vi "Pendulum7_0.vi"() -> ()   [LabVIEW 2021]
uses:
  <vilib>/Utility/miscctls.llb/LVBoundsTypeDef.ctl
  <vilib>/Platform/TimedLoop/XDataNode/timing_clust.ctl
  <vilib>/Platform/TimedLoop/XDataNode/nitl_modes.ctl
  <vilib>/Platform/TimedLoop/XDataNode/wakeup.ctl
  <vilib>/platform/TimedLoop/XDataNode/XDataNode.xnode
  <vilib>/Platform/TimedLoop/XDataNode/XDNodeRunTimeDep.lvlib
panel:
  out "error out":errorcluster
  in  "Enum 2":enum16{"stop", "start"}(ring)
  out "L":dbl
  out "Waveform Graph 2":waveform(dbl)(graph)
  in  "Остановить симуляцию":bool
  in  "Начать симуляцию":bool
  out "Object":bool
  in  "Cieling":bool
  in  "Начальная амплитуда":dbl
  in  "Амплитуда":dbl
  in  "Угловая частота внешней силы":dbl min=0.0
  in  "Вязкость среды":dbl min=0.0
  in  "Масса":dbl min=0.0 max=3000.0
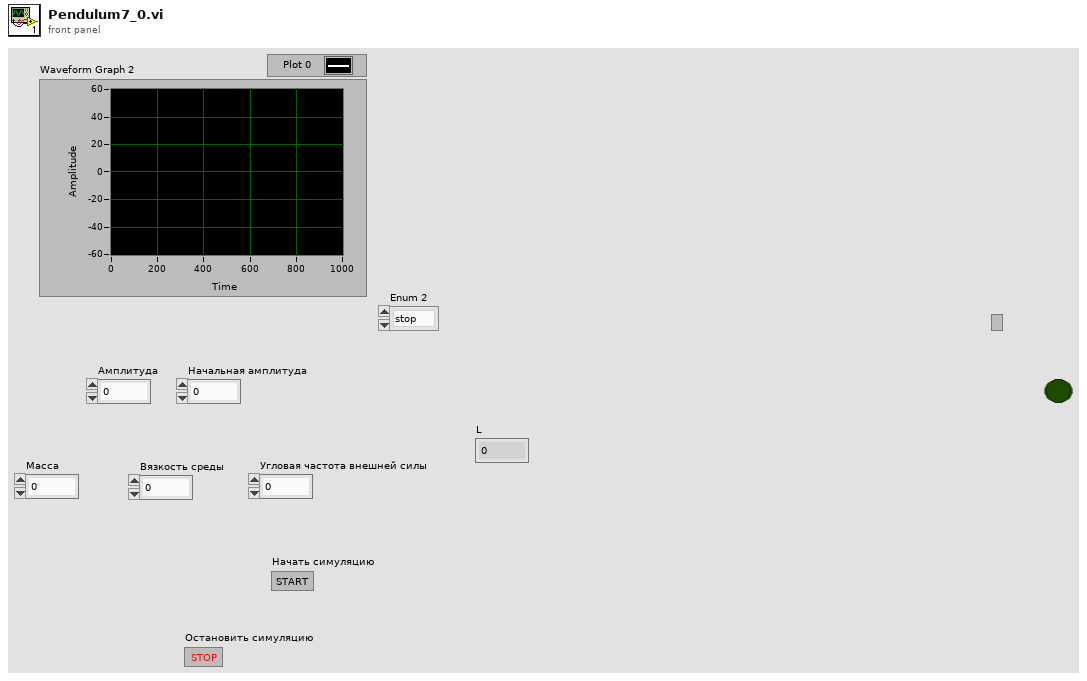
[diagram p1: front panel]
types:
  T1 = typedef "XDNodeRunTimeDep.lvlib/timing_clust.ctl" = cluster{"Expected End [f-1]":u64, "Actual End [f-1]":u64, "Finished Late? [f-1]":bool, "Expected End [i-1]":u64, "Actual End [i-1]":u64, "Finished Late? [i-1]":bool, "Expected Start [i]":u64, "Actual Start [i]":u64, "Expected Start [f]":u64, "Actual Start [f]":u64, "Source Name":string, "Structure Name":string, "Period":i64, "Deadline":i64, "Offset":i64, "Start":i64, "Priority":i32, "Timeout":i32, "Mode":T2, "Wakeup Reason":T3, "Error":errorcluster, "Source Type":string, "Secondary Source Type":string, "Global End Time":u64, "Global Start Time":u64, "Frame Duration":u64, "Iteration Duration":u64, "Assigned CPU":i32, "I/O Scan Engine Mode":u32}
  T2 = typedef "XDNodeRunTimeDep.lvlib/nitl_modes.ctl" = enum32{"No Change", "Process missed periods, maintain original phase", "Discard missed periods, maintain original phase", "Process missed periods, ignore original phase", "Discard missed periods, ignore original phase"}
  T3 = typedef "XDNodeRunTimeDep.lvlib/wakeup.ctl" = enum32{"Normal", "Aborted", "Asynchronous wakeup", "Timing source error", "Timed loop error", "Timeout"}
  T4 = typedef "LVBoundsTypeDef.ctl" = cluster{"Width":u32, "Height":u32}
  T5 = typedef "LVPoint32TypeDef.ctl" = cluster{"Horizontal":i32, "Vertical":i32}
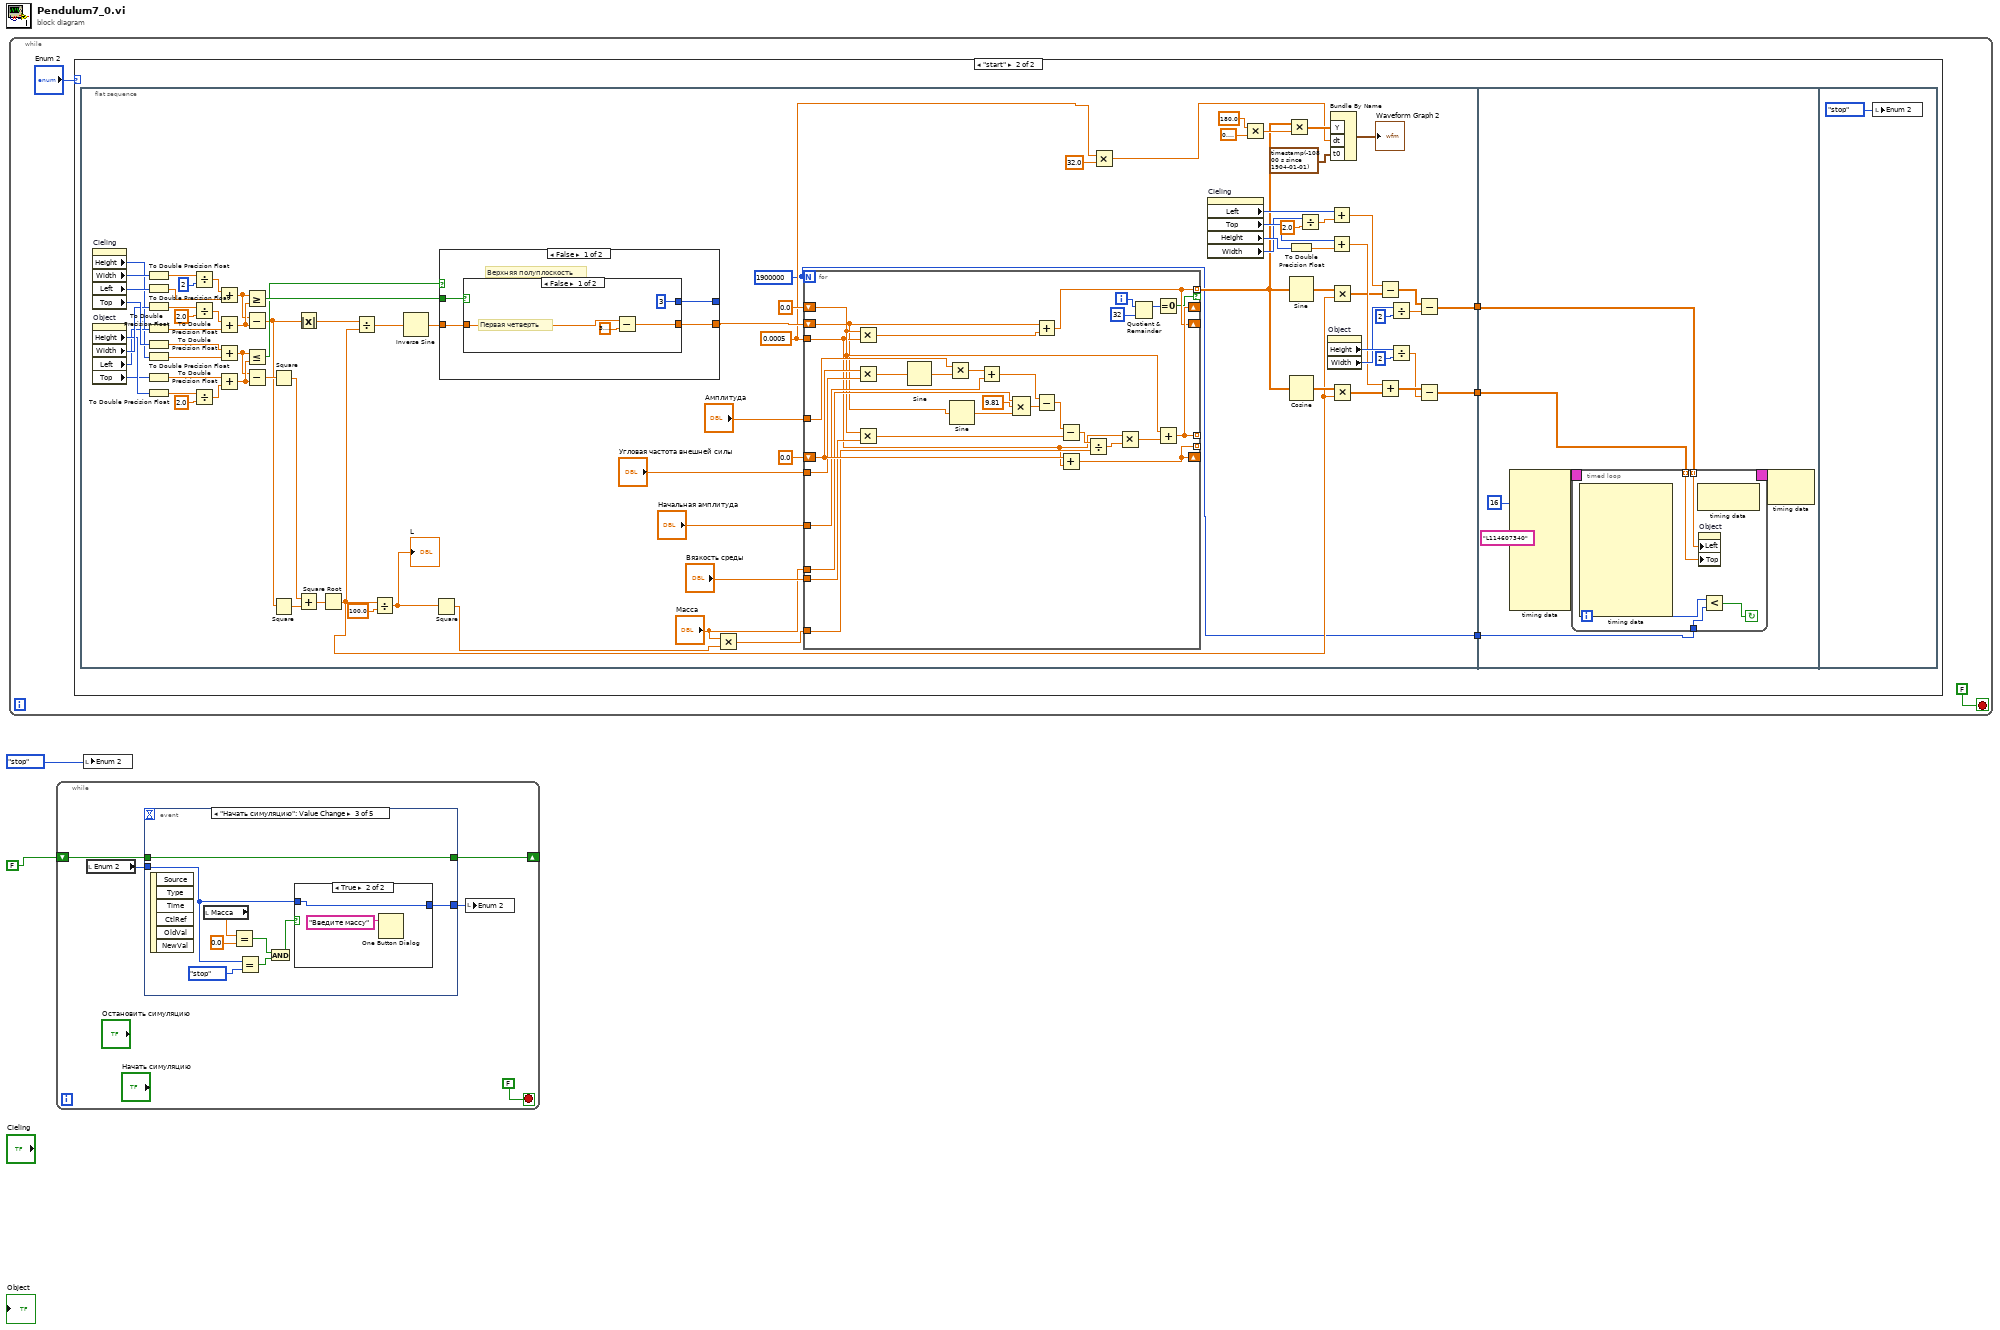
[diagram p0: block diagram]
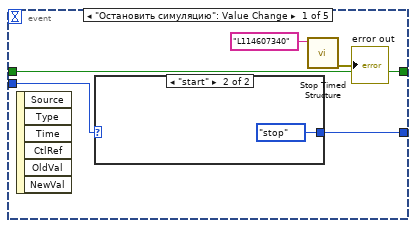
[diagram p2: hidden frame]
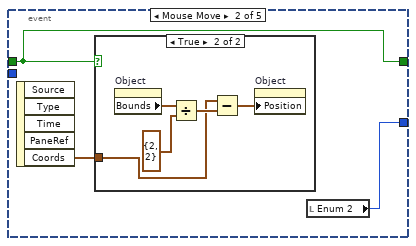
[diagram p4: hidden frame]
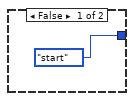
[diagram p6: hidden frame]
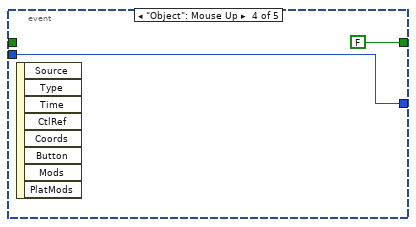
[diagram p7: hidden frame]
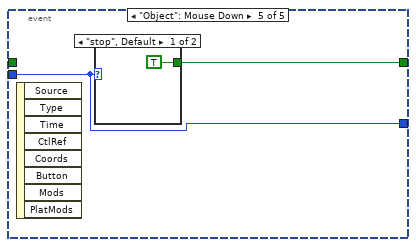
[diagram p8: hidden frame]
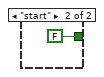
[diagram p9: hidden frame]
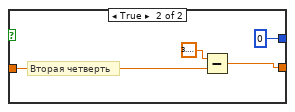
[diagram p11: hidden frame]
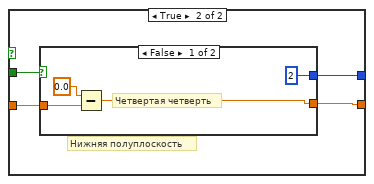
[diagram p12: hidden frame]
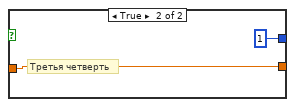
[diagram p13: hidden frame]
diagram:
  n1 = while {
    stop <- FALSE stop-if-true
    n2 = case shown="\"start\"" "Enum 2" {
      frame "stop", Default {
      }
      frame "start" {
        n3 = flat-sequence {
          tunnel: [w22] -> w7
          tunnel: [w21] -> w6
          tunnel: [w8] -> w5
          tunnel: w7 -> [w144]
          tunnel: w6 -> [w146]
          tunnel: w5 -> [w145]
          frame #0 {
            w8 = 1900000
            w9 = 0.0005 ("Real")
            n4 = property on="Cieling" class="Bool"() -> ("Height"=w66:u32, "Width"=w80:u32, "Left"=w78:i32, "Top"=w76:i32)  [unwired: 2 in, 2 out]
            n5 = property on="Object" class="Bool (strict)"() -> ("Height"=w73:u32, "Width"=w74:u32, "Left"=w71:i32, "Top"=w70:i32)  [unwired: 2 in, 2 out]
            n6 = To Double Precision Float(number=w80) -> (double precision float=w81:dbl)
            n7 = To Double Precision Float(number=w78) -> (double precision float=w79:dbl)
            n8 = To Double Precision Float(number=w74) -> (double precision float=w75:dbl)
            n9 = To Double Precision Float(number=w71) -> (double precision float=w72:dbl)
            n10 = To Double Precision Float(number=w76) -> (double precision float=w77:dbl)
            n11 = To Double Precision Float(number=w66) -> (double precision float=w65:dbl)
            n12 = To Double Precision Float(number=w70) -> (double precision float=w90:dbl)
            n13 = To Double Precision Float(number=w73) -> (double precision float=w82:dbl)
            n14 = Divide(x=w81, y=u32 2) -> (x/y=w68:dbl)
            n15 = Divide(x=w75, y=2.0) -> (x/y=w67:dbl)
            n16 = Divide(x=w82, y=2.0) -> (x/y=w83:dbl)
            n17 = Add(x=w68, y=w79) -> (x+y=w85:dbl)
            n18 = Add(x=w67, y=w72) -> (x+y=w86:dbl)
            n19 = Add(x=w77, y=w65) -> (x+y=w87:dbl)
            n20 = Add(x=w90, y=w83) -> (x+y=w88:dbl)
            n21 = Greater Or Equal?(x=w85, y=w86) -> (x >= y?=w84:bool)
            n22 = Subtract(x=w85, y=w86) -> (x-y=w63:dbl)
            n23 = Less Or Equal?(x=w87, y=w88) -> (x <= y?=w69:bool)
            n24 = Subtract(x=w87, y=w88) -> (x-y=w64:dbl)
            n25 = Square(x=w64) -> (x^2=w51:dbl)
            n26 = Square(x=w63) -> (x^2=w50:dbl)
            n27 = Absolute Value(x=w63) -> (abs(x)=w62:dbl)
            n28 = Add(x=w51, y=w50) -> (x+y=w52:dbl)
            n29 = Square Root(x=w52) -> (sqrt(x)=w12:dbl)
            n30 = Divide(x=w62, y=w12) -> (x/y=w53:dbl)
            n31 = Divide(x=w12, y=100.0) -> (x/y=w11:dbl)
            "L" <- w11
            n32 = Inverse Sine(1:w53) -> (0:w89:dbl)
            n33 = Square(x=w11) -> (x^2=w56:dbl)
            n34 = case shown="False" w69 {
              tunnel: [w94 w106] -> _
              tunnel: w84 -> [w92 w105]
              tunnel: w89 -> [w93 w104]
              tunnel: [w91 w103] -> w10
              frame False {
                # "Верхняя полуплоскость"
                n35 = case shown="False" w92 {
                  tunnel: [3 0] -> w94
                  tunnel: [w96 w100] -> w91
                  tunnel: w93 -> [w95 w99]
                  frame False {
                    # "Первая четверть"
                    n36 = Subtract(x=w95, y=3.141592653589793) -> (x-y=w96:dbl)
                  }
                  frame True {
                    # "Вторая четверть"
                    n37 = Subtract(x=3.141592653589793, y=w99) -> (x-y=w100:dbl)
                  }
                }
              }
              frame True {
                # "Нижняя полуплоскость"
                n38 = case shown="False" w105 {
                  tunnel: [2 ("index") 1 ("index")] -> w106
                  tunnel: w104 -> [w107 w111]
                  tunnel: [w108 w111] -> w103
                  frame False {
                    # "Четвертая четверть"
                    n39 = Subtract(x=0.0, y=w107) -> (x-y=w108:dbl)
                  }
                  frame True {
                    # "Третья четверть"
                  }
                }
              }
            }
            n40 = Multiply(x="Масса", y=w56) -> (x*y=w55:dbl)
            n41 = for {
              N: w8 -> [_]
              shift-right: [w142] -> _
              shift-left: 0.0 ("Real") -> [w122]
              tunnel: [w142] -> _ mode=indexing
              tunnel: w9 -> [w121]
              shift-right: [w123] -> _
              shift-left: 0.0 ("Угловая частота внешней силы") -> [w140]
              tunnel: "Угловая частота внешней силы" -> [w139]
              tunnel: "Амплитуда" -> [w136]
              tunnel: "Начальная амплитуда" -> [w134]
              tunnel: "Масса" -> [w131]
              shift-right: [w118] -> _
              shift-left: w10 -> [w113]
              tunnel: "Вязкость среды" -> [w128]
              tunnel: w55 -> [w125]
              tunnel: [w123] -> _ mode=indexing
              tunnel: [w118] -> w15 mode=indexing if=w114
              i -> [w117]
              n42 = Multiply(x=w122, y=w121) -> (x*y=w120:dbl)
              n43 = Multiply(x=w140, y=w139) -> (x*y=w138:dbl)
              n44 = Multiply(x=w122, y=w128) -> (x*y=w127:dbl)
              n45 = Sine(x=w138) -> (sin(x)=w137:dbl)
              n46 = Multiply(x=w136, y=w137) -> (x*y=w135:dbl)
              n47 = Sine(x=w113) -> (sin(x)=w130:dbl)
              n48 = Add(x=w135, y=w134) -> (x+y=w133:dbl)
              n49 = Compound Arithmetic op=MULTIPLY(w131, 9.81 ("value"), w130) -> (w129:dbl)
              n50 = Add(x=w113, y=w120) -> (x+y=w118:dbl)
              n51 = Subtract(x=w133, y=w129) -> (x-y=w132:dbl)
              n52 = Subtract(x=w132, y=w127) -> (x-y=w126:dbl)
              n53 = Add(x=w140, y=w121) -> (x+y=w123:dbl)
              n54 = Divide(x=w126, y=w125) -> (x/y=w124:dbl)
              n55 = Multiply(x=w121, y=w124) -> (x*y=w141:dbl)
              n56 = Quotient & Remainder(x=w117, y=32) -> (x-y*floor(x/y)=w115:i32)  [unwired: 1 out]
              n57 = Equal To 0?(x=w115) -> (x = 0?=w114:bool)
              n58 = Add(x=w122, y=w141) -> (x+y=w142:dbl)
            }
            n59 = Multiply(x=w9, y=32.0) -> (x*y=w13:dbl)
            n60 = property on="Cieling" class="Bool"() -> ("Left"=w38:i32, "Top"=w36:i32, "Height"=w25:u32, "Width"=w24:u32)  [unwired: 2 in, 2 out]
            n61 = Multiply(x=180.0, y=0.3183098861837907) -> (x*y=w17:dbl)
            n62 = Multiply(x=w15, y=w17) -> (x*y=w16:dbl[])
            n63 = To Double Precision Float(number=w25) -> (double precision float=w35:dbl)
            n64 = Sine(x=w15) -> (sin(x)=w41:dbl[])
            n65 = Cosine(x=w15) -> (cos(x)=w42:dbl[])
            n66 = Divide(x=w24, y=2.0) -> (x/y=w37:dbl)
            n67 = property on="Object" class="Bool (strict)"() -> ("Height"=w33:u32, "Width"=w32:u32)  [unwired: 2 in, 2 out]
            n68 = Add(x=w38, y=w37) -> (x+y=w28:dbl)
            n69 = Add(x=w36, y=w35) -> (x+y=w29:dbl)
            n70 = Bundle By Name("Y"=w16, "dt"=w13, "t0"=timestamp(-10800 s since 1904-01-01)) -> (→"Waveform Graph 2":waveform(dbl))  [unwired: 1 in]
            n71 = Multiply(x=w41, y=w12) -> (x*y=w26:dbl[])
            n72 = Multiply(x=w42, y=w12) -> (x*y=w27:dbl[])
            n73 = Subtract(x=w28, y=w26) -> (x-y=w39:dbl[])
            n74 = Add(x=w29, y=w27) -> (x+y=w40:dbl[])
            n75 = Divide(x=w32, y=u32 2) -> (x/y=w30:dbl)
            n76 = Divide(x=w33, y=u32 2) -> (x/y=w31:dbl)
            n77 = Subtract(x=w39, y=w30) -> (x-y=w22:dbl[])
            n78 = Subtract(x=w40, y=w31) -> (x-y=w21:dbl[])
          }
          frame #1 {
            n79 = node-c288(i64 16 ("Period"), "L114607340" ("Structure Name")) -> (w149:T1)  [unwired: 8 in]
            n80 = timed-loop {
              timing: w149 -> [_]
              timing-out: [_] -> w148
              tunnel: w146 -> [w154] mode=indexing
              tunnel: w145 -> [w152]
              tunnel: w144 -> [w150] mode=indexing
              i -> [w153]
              stop <- w151 continue-if-true
              n81 = node-c288() -> ()  [unwired: 1 in, 10 out]
              n82 = node-c288() -> ()  [unwired: 1 in, 1 out]
              n83 = property on="Object" class="Bool (strict)"("Left"=w150, "Top"=w154) -> ()  [unwired: 2 in, 2 out]
              n84 = Less?(x=w153, y=w152) -> (x < y?=w151:bool)
            }
            n85 = node-c288(w148) -> ()  [unwired: 1 out]
          }
          frame #2 {
            n86 = local write "Enum 2"(enum16{"stop", "start"}."stop" ("Enum")) -> ()
          }
        }
      }
    }
  }
  n87 = while {
    shift-right: [w164] -> _
    shift-left: FALSE -> [w165]
    stop <- FALSE stop-if-true
    n88 = local read "Enum 2"() -> (w163:enum16{"stop", "start"})
    n89 = event shown="[2] \"Начать симуляцию\": Value Change" {
      selector: _ -> [_ _ _ _ _]
      dyn-events: _ -> [_ _ _ _ _]
      timeout: _ -> [_ _ _ _ _]
      tunnel: [w171 w175 w188 w195 w198] -> w166
      tunnel: w163 -> [w170 _ w186 w195 w198]
      tunnel: [w172 w176 w191 FALSE w197] -> w164
      tunnel: w165 -> [w172 w176 w191 _ _]
      event "Остановить симуляцию": Value Change {
        n90 = event-data() -> ()  [unwired: 1 in, 6 out]
        n91 = case shown="\"start\"" w170 {
          selector: w170 -> [w173 _]
          tunnel: [w173 enum16{"stop", "start"}."stop" ("Enum")] -> w171
          frame "stop", Default {
          }
          frame "start" {
          }
        }
        n92 = call <vilib>:"Stop Timed Structure.vi"("name"="L114607340") -> ("error out"=→"error out":errorcluster)  [unwired: 10 in]
      }
      event Mouse Move {
        n93 = event-data() -> ("Coords"=w177:T5)  [unwired: 1 in, 4 out]
        n94 = case shown="True" w176 {
          tunnel: w177 -> [_ w179]
          frame False {
          }
          frame True {
            n95 = property on="Object" class="Bool (strict)"() -> ("Bounds"=w182:T4)  [unwired: 2 in, 2 out]
            n96 = Divide(x=w182, y=T4 {"Width"=2, "Height"=2}) -> (x/y=w180:cluster{"Width":dbl, "Height":dbl})
            n97 = Subtract(x=w179, y=w180) -> (x-y=w181:cluster{dbl, dbl})
            n98 = property on="Object" class="Bool (strict)"("Position"=w181) -> ()  [unwired: 2 in, 2 out]
          }
        }
        n99 = local read "Enum 2"() -> (w175:enum16{"stop", "start"})
      }
      event "Начать симуляцию": Value Change {
        n100 = event-data() -> ()  [unwired: 1 in, 6 out]
        n101 = local read "Масса"() -> (w190:dbl)
        n102 = Equal?(x=w190, y=0.0) -> (x = y?=w184:bool)
        n103 = Equal?(x=w186, y=enum16{"stop", "start"}."stop" ("Enum")) -> (x = y?=w185:bool)
        n104 = And(x=w184, y=w185) -> (x .and. y?=w183:bool)
        n105 = case shown="True" w183 {
          tunnel: w186 -> [_ w193]
          tunnel: [enum16{"stop", "start"}."start" ("Enum") w193] -> w188
          frame False {
          }
          frame True {
            n106 = One Button Dialog(message="Введите массу") -> ()  [unwired: 1 in, 1 out]
          }
        }
      }
      event "Object": Mouse Up {
        n107 = event-data() -> ()  [unwired: 1 in, 8 out]
      }
      event "Object": Mouse Down {
        n108 = event-data() -> ()  [unwired: 1 in, 8 out]
        n109 = case shown="\"stop\", Default" w198 {
          tunnel: [TRUE FALSE] -> w197
          frame "stop", Default {
          }
          frame "start" {
          }
        }
      }
    }
    n110 = local write "Enum 2"(w166) -> ()
  }
  n111 = local write "Enum 2"(enum16{"stop", "start"}."stop" ("Enum 2")) -> ()
